vi "Define_Index_of_Lowest_Cost_in_Subtrack_Row-1.vi"(3 "[IN] Cost functions":i8[](array[numeric]), 6 "[IN] Subtracks in Row":T1(array[cluster])) -> (1 "[OUT] Index of Optimal Subtrack":i32)   [LabVIEW 2017]
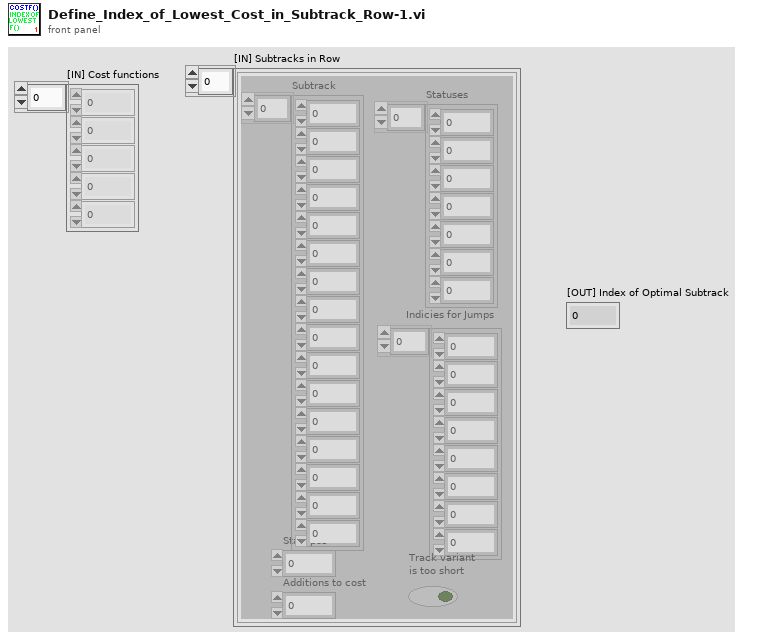
[diagram p1: front panel]
types:
  T1 = cluster{"Subtrack":dbl[], "Statuses":i16[], "Start pos":i32, "Additions to cost":i8, "Track variant \nis too short":bool, "Indicies for Jumps":i32[]}[]
  T2 = cluster{"Subtrack":dbl[], "Statuses":i16[], "Start pos":i32, "Additions to cost":i8, "Track variant \nis too short":bool, "Indicies for Jumps":i32[]}
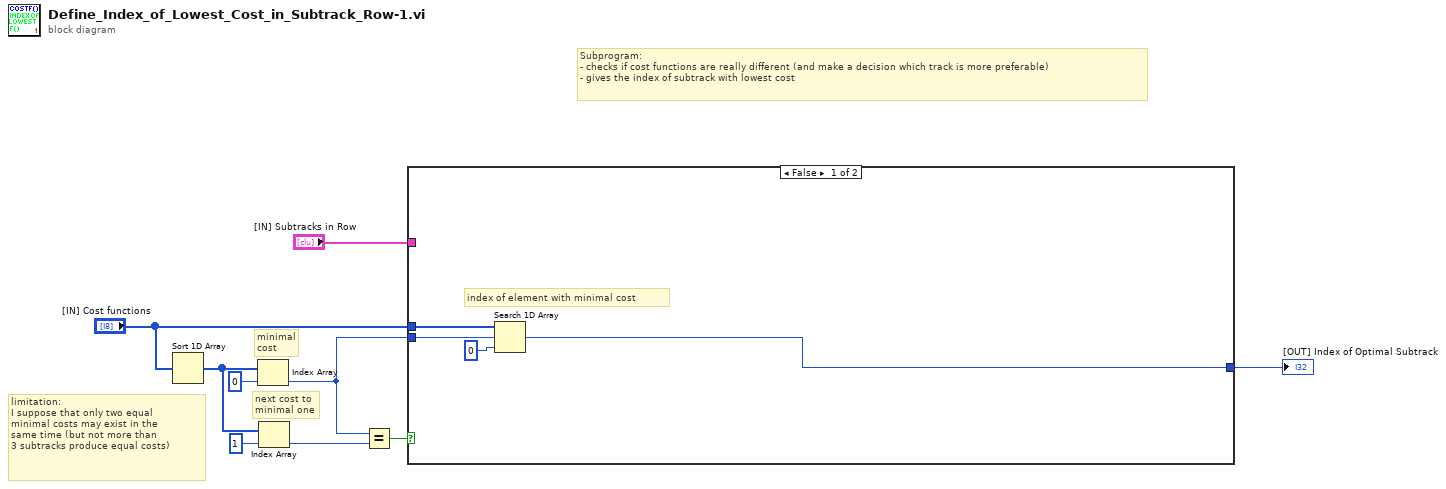
[diagram p0: block diagram]
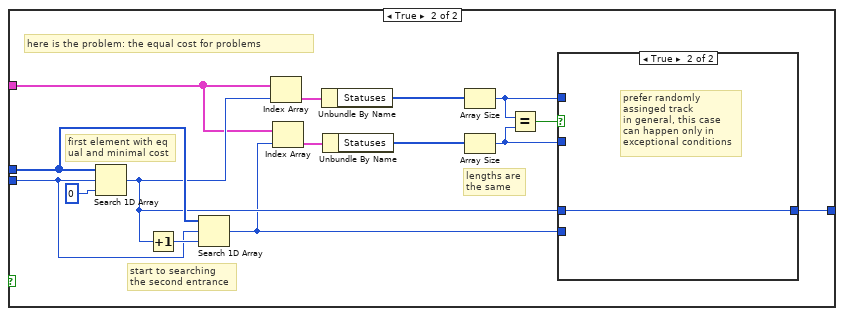
[diagram p2: hidden frame]
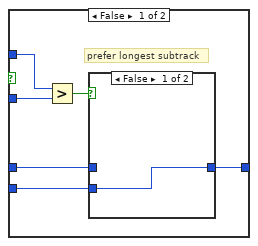
[diagram p3: hidden frame]
diagram:
  # "limitation: \nI suppose that only two equal\nminimal costs may exist in the \nsame time (but not more than\n3 subtracks produce equal costs)"
  # "next cost to \nminimal one"
  # "minimal\ncost"
  # "Subprogram:\n- checks if cost functions are really different (and make a decision which track is more preferable)\n- gives the index of subtrack with lowest cost"
  n1 = Sort 1D Array(array="[IN] Cost functions") -> (sorted array=w5:i8[])
  n2 = Index Array(array=w5, index=0) -> (element=w4:i8)
  n3 = Index Array(array=w5, index=1) -> (element=w7:i8)
  n4 = Equal?(x=w4, y=w7) -> (x = y?=w6:bool)
  n5 = case shown="False" w6 {
    tunnel: "[IN] Cost functions" -> [w12 w24]
    tunnel: w4 -> [w11 w26]
    tunnel: [w10 w14] -> w1
    tunnel: "[IN] Subtracks in Row" -> [_ w18]
    frame False {
      # "index of element with minimal cost"
      n6 = Search 1D Array(1D array=w12, element=w11, start index (0)=0) -> (index of element=w10:i32)
    }
    frame True {
      # "lengths are\nthe same"
      # "start to searching\nthe second entrance"
      # "first element with eq\nual and minimal cost"
      # "here is the problem: the equal cost for problems"
      n7 = Search 1D Array(1D array=w24, element=w26, start index (0)=0) -> (index of element=w21:i32)
      n8 = Increment(x=w21) -> (x+1=w27:i32)
      n9 = Search 1D Array(1D array=w24, element=w26, start index (0)=w27) -> (index of element=w17:i32)
      n10 = Index Array(array=w18, index=w21) -> (element=w20:T2)
      n11 = Index Array(array=w18, index=w17) -> (element=w16:T2)
      n12 = Unbundle By Name(w20) -> ("Statuses"=w19:i16[])
      n13 = Unbundle By Name(w16) -> ("Statuses"=w15:i16[])
      n14 = Array Size(array=w19) -> (size(s)=w23:i32)
      n15 = Array Size(array=w15) -> (size(s)=w22:i32)
      n16 = Equal?(x=w23, y=w22) -> (x = y?=w25:bool)
      n17 = case shown="True" w25 {
        tunnel: w17 -> [w31 _]
        tunnel: w21 -> [w30 w37]
        tunnel: w23 -> [w34 _]
        tunnel: w22 -> [w33 _]
        tunnel: [w29 w37] -> w14
        frame False {
          # "prefer longest subtrack"
          n18 = Greater?(x=w34, y=w33) -> (0:w32:bool)
          n19 = case shown="False" w32 {
            tunnel: w31 -> [w35 _]
            tunnel: w30 -> [_ w36]
            tunnel: [w35 w36] -> w29
            frame False {
            }
            frame True {
            }
          }
        }
        frame True {
          # "prefer randomly \nassinged track\nin general, this case\ncan happen only in \nexceptional conditions"
        }
      }
    }
  }
  "[OUT] Index of Optimal Subtrack" <- w1
